vi "Data to Waveform.vi"(8 "error in":errorcluster, 11 "DIG_IO in":refnum<class "DIG_IO.lvclass">) -> (0 "error out":errorcluster, 3 "DIG_IO out":refnum<class "DIG_IO.lvclass">)   [LabVIEW 2019, in "DIG_IO.lvlib" / "DIG_IO.lvclass"]
uses:
  Library/DIG_IO.lvclass
  C:/Users/Public/Documents/Development/builds/Instruments/Instruments.lvlibp/Library/Instruments.lvclass
  Library/DIG_IO.lvclass/DIG_IO.ctl
  builds/Instruments/Instruments.lvlibp/Accessors/Write Measured.vi
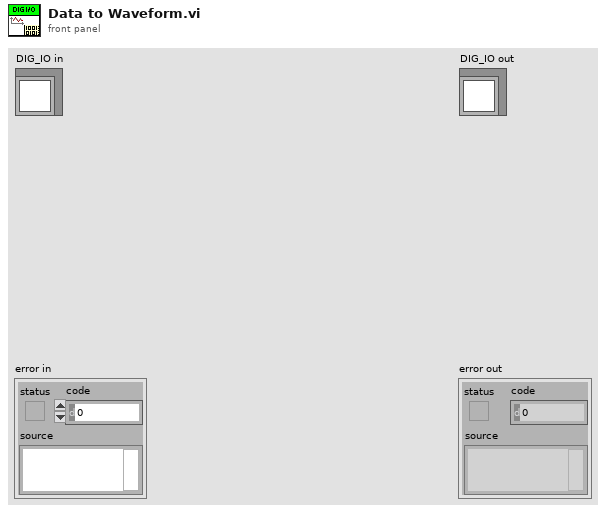
[diagram p1: front panel]
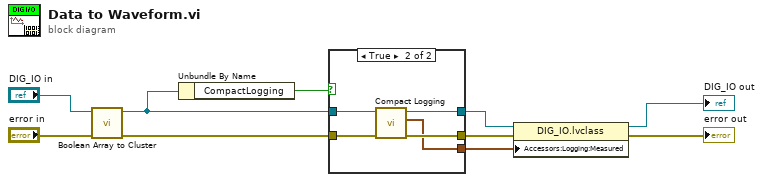
[diagram p0: block diagram]
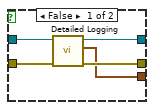
[diagram p2: hidden frame]
diagram:
  n1 = call "Boolean Array to Cluster.vi"("error in"="error in", "DIG_IO in"="DIG_IO in") -> ("error out"=w5:errorcluster, "DIG_IO out"=w4:refnum<class "DIG_IO.lvclass">)  [unwired: 8 in]
  n2 = Unbundle By Name(w4) -> ("CompactLogging"=w6:bool)
  n3 = case shown="True" w6 {
    tunnel: w5 -> [w14 w20]
    tunnel: w4 -> [w15 w19]
    tunnel: [w13 w18] -> w3
    tunnel: [w12 w17] -> w2
    tunnel: [w11 w16] -> w1
    frame False {
      n4 = call "Detailed Logging.vi"("error in"=w14, "DIG_IO in"=w15) -> ("error out"=w12:errorcluster, "Detailed Record"=w11:waveform(i16)[], "DIG_IO out"=w13:refnum<class "DIG_IO.lvclass">)  [unwired: 7 in]
    }
    frame True {
      n5 = call "Compact Logging.vi"("error in"=w20, "DIG_IO in"=w19) -> ("error out"=w17:errorcluster, "Compact Record"=w16:waveform(i16)[], "DIG_IO out"=w18:refnum<class "DIG_IO.lvclass">)  [unwired: 7 in]
    }
  }
  n6 = property class="DIG_IO.lvclass"(reference=w3, error in=w2, "Accessors:Logging:Measured"=w1) -> (reference out=→"DIG_IO out":refnum<class "DIG_IO.lvclass">, error out=→"error out":errorcluster)
